vi "Main Dialog.vi"() -> ()   [LabVIEW 2020, in "Process Generation.lvlib" / "New Class Dialog.lvclass"]
uses:
  New Class Dialog.lvclass
  Tag Tree Helper/Tag Tree Helper.lvclass
  Process Generator/Process Generator.lvclass
panel:
  in  "Parent Class":string(tree)
  in  "Process Name":string
  in  "Save to Folder":path
  in  "Commit":bool
  in  "Cancel":bool
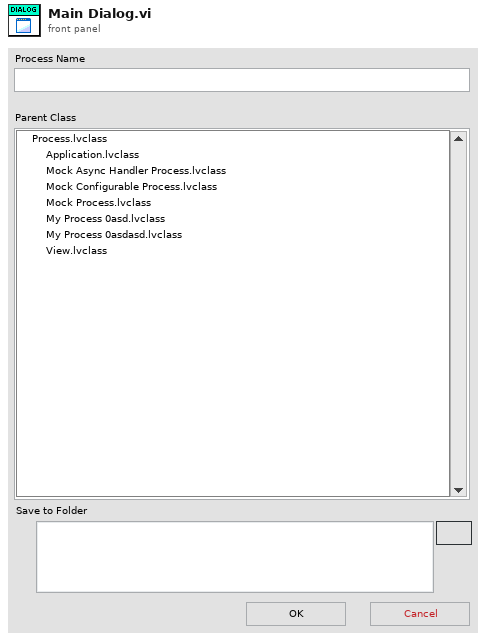
[diagram p1: front panel]
types:
  T1 = enum8{"Enabled", "Disabled", "Disabled and Grayed Out"}
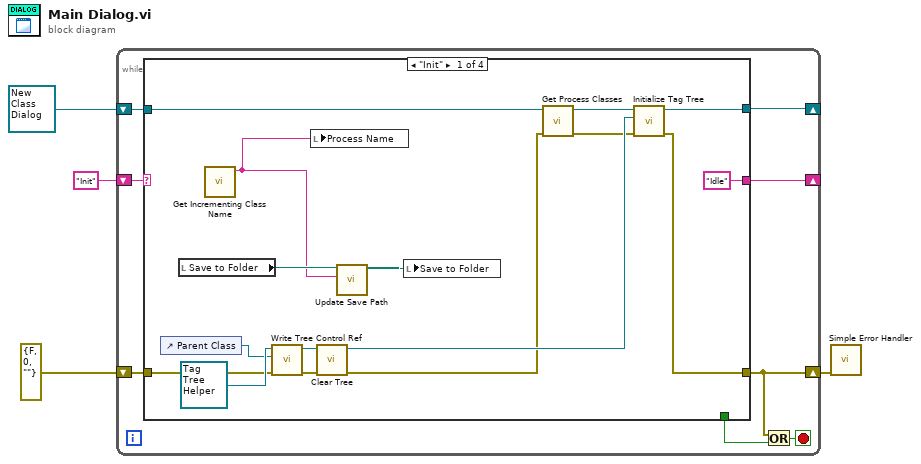
[diagram p0: block diagram]
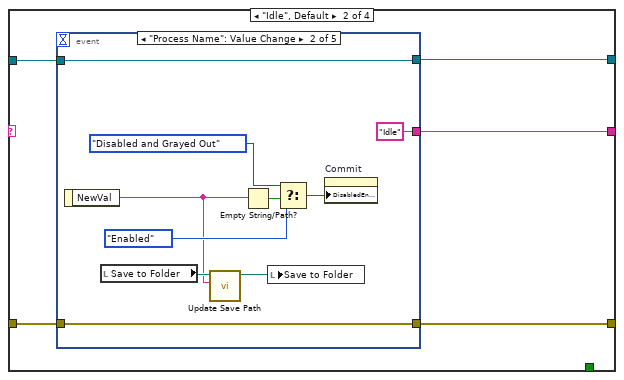
[diagram p2: hidden frame]
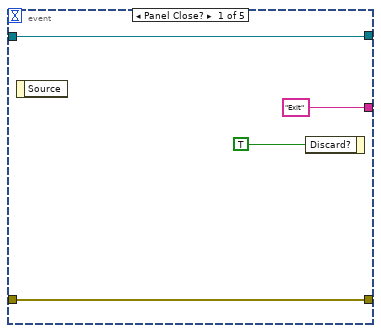
[diagram p3: hidden frame]
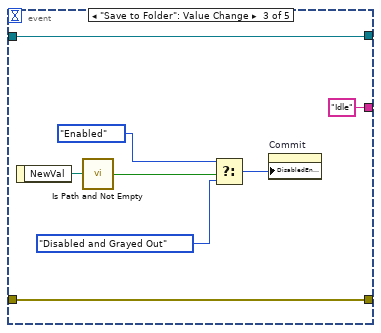
[diagram p4: hidden frame]
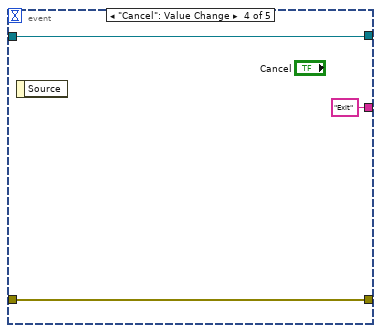
[diagram p5: hidden frame]
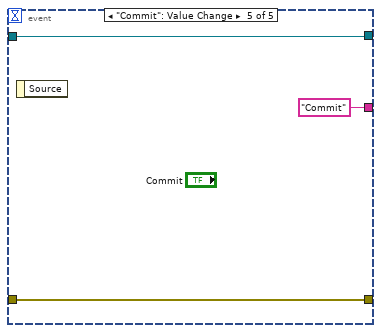
[diagram p6: hidden frame]
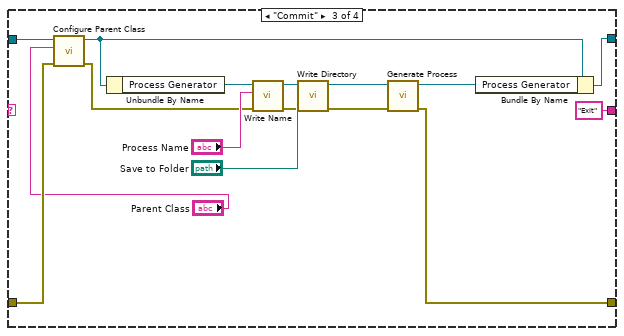
[diagram p7: hidden frame]
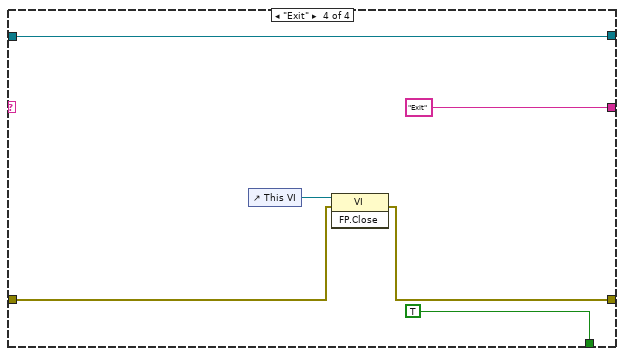
[diagram p8: hidden frame]
diagram:
  n1 = while {
    shift-right: [w9] -> _
    shift-left: refnum<class "New Class Dialog.lvclass"> refnum ("New Class Dialog In") -> [w10]
    shift-right: [w5] -> w2
    shift-left: errorcluster {"status"=FALSE, "code"=0, "source"=""} ("error in (no error)") -> [w11]
    shift-right: [w8] -> _
    shift-left: "Init" -> [w12]
    stop <- w6 stop-if-true
    n2 = case shown="\"Init\"" w12 {
      tunnel: [w22 w33 w64 w79] -> w5
      tunnel: w11 -> [w19 w32 w71 w78]
      tunnel: w10 -> [w27 w31 w68 w83]
      tunnel: [w24 w30 w70 w83] -> w9
      tunnel: ["Idle" w29 "Exit" "Exit"] -> w8
      tunnel: [_ _ _ TRUE] -> w7
      frame "Init" {
        n3 = control-ref of="Parent Class"() -> (w25:refnum<vi>)
        n4 = local read "Save to Folder"() -> (w17:path)
        n5 = call "Get Incrementing Class Name.vi"() -> ("String"=w16:string)  [unwired: 11 in]
        n6 = call "Write Tree Control Ref.vi"("error in (no error)"=w19, "Tag Tree Reference"=w25, "Tag Tree Helper In"=refnum<class "Tag Tree Helper.lvclass"> refnum ("Support Utilities.lvlib:Tag Tree.lvclass")) -> ("error out"=w23:errorcluster, "Tag Tree Helper Out"=w20:refnum<class "Tag Tree Helper.lvclass">)  [unwired: 7 in]
        n7 = local write "Process Name"(w16) -> ()
        n8 = call "Clear Tree.vi"("error in (no error)"=w23, "Tag Tree Helper In"=w20) -> ("error out"=w18:errorcluster, "Tag Tree Helper Out"=w21:refnum<class "Tag Tree Helper.lvclass">)  [unwired: 8 in]
        n9 = call "Update Save Path.vi"("Process Name"=w16, "Current Path"=w17) -> ("Updated Path"=w15:path)  [unwired: 9 in]
        n10 = local write "Save to Folder"(w15) -> ()
        n11 = call "Get Process Classes.vi"("error in (no error)"=w18, "New Class Dialog In"=w27) -> ("error out"=w13:errorcluster, "New Class Dialog Out"=w14:refnum<class "New Class Dialog.lvclass">)  [unwired: 8 in]
        n12 = call "Initialize Tag Tree.vi"("error in (no error)"=w13, "Tag Tree Helper"=w21, "New Class Dialog In"=w14) -> ("error out"=w22:errorcluster, "New Class Dialog Out"=w24:refnum<class "New Class Dialog.lvclass">)  [unwired: 7 in]
      }
      frame "Idle", Default {
        n13 = event shown="[1] \"Process Name\": Value Change" {
          selector: _ -> [_ _ _ _ _]
          dyn-events: _ -> [_ _ _ _ _]
          timeout: _ -> [_ _ _ _ _]
          tunnel: [w37 w47 w55 w57 w61] -> w33
          tunnel: w32 -> [w37 w47 w55 w57 w61]
          tunnel: w31 -> [w36 w46 w54 w58 w60]
          tunnel: [w36 w46 w54 w58 w60] -> w30
          tunnel: ["Exit" "Idle" "Idle" "Exit" "Commit"] -> w29
          event Panel Close? {
            n14 = event-data() -> ()  [unwired: 1 in, 1 out]
            n15 = event-data("Discard?"=TRUE) -> ()  [unwired: 1 in, 1 out]
          }
          event "Process Name": Value Change {
            n16 = event-data() -> ("NewVal"=w38:string)  [unwired: 1 in]
            n17 = local read "Save to Folder"() -> (w39:path)
            n18 = call "Update Save Path.vi"("Process Name"=w38, "Current Path"=w39) -> ("Updated Path"=w40:path)  [unwired: 9 in]
            n19 = Empty String/Path?(string/path=w38) -> (empty?=w45:bool)
            n20 = local write "Save to Folder"(w40) -> ()
            n21 = Select(t=T1."Disabled and Grayed Out" ("Disabled"), s=w45, f=T1."Enabled") -> (s? t:f=w42:T1)
            n22 = property on="Commit" class="Bool"("DisabledEnum"=w42) -> ()  [unwired: 2 in, 2 out]
          }
          event "Save to Folder": Value Change {
            n23 = event-data() -> ("NewVal"=w53:path)  [unwired: 1 in]
            n24 = call <vilib>:"Is Path and Not Empty.vi"("path"=w53) -> ("Is Path and Not Empty?"=w52:bool)  [unwired: 4 in]
            n25 = Select(t=T1."Enabled" ("f"), s=w52, f=T1."Disabled and Grayed Out" ("Disabled")) -> (s? t:f=w49:T1)
            n26 = property on="Commit" class="Bool"("DisabledEnum"=w49) -> ()  [unwired: 2 in, 2 out]
          }
          event "Cancel": Value Change {
            n27 = event-data() -> ()  [unwired: 1 in, 1 out]
          }
          event "Commit": Value Change {
            n28 = event-data() -> ()  [unwired: 1 in, 1 out]
          }
        }
      }
      frame "Commit" {
        n29 = call "Configure Parent Class.vi"("error in (no error)"=w71, "Parent Class"="Parent Class", "New Class Dialog In"=w68) -> ("error out"=w69:errorcluster, "New Class Dialog Out"=w67:refnum<class "New Class Dialog.lvclass">)  [unwired: 7 in]
        n30 = Unbundle By Name(w67) -> ("Process Generator"=w74:refnum<class "Process Generator.lvclass">)
        n31 = call "Write Name.vi"("error in (no error)"=w69, "Name"="Process Name", "Process Generator In"=w74) -> ("error out"=w72:errorcluster, "Process Generator Out"=w73:refnum<class "Process Generator.lvclass">)  [unwired: 7 in]
        n32 = call "Write Directory.vi"("error in (no error)"=w72, "Directory"="Save to Folder", "Process Generator in"=w73) -> ("error out"=w62:errorcluster, "Process Generator out"=w63:refnum<class "Process Generator.lvclass">)  [unwired: 7 in]
        n33 = call "Generate Process.vi"("error in (no error)"=w62, "Process Generator In"=w63) -> ("error out"=w64:errorcluster, "Process Generator Out"=w65:refnum<class "Process Generator.lvclass">)  [unwired: 8 in]
        n34 = Bundle By Name(cluster=w67, "Process Generator"=w65) -> (w70:refnum<class "New Class Dialog.lvclass">)
      }
      frame "Exit" {
        n35 = control-ref of="This VI"() -> (w80:refnum<vi>)
        n36 = invoke class="VI" method="FP.Close"(reference=w80, error in=w78) -> (error out=w79:errorcluster)  [unwired: 1 in, 2 out]
      }
    }
    n37 = Or(x=w5, y=w7) -> (x .or. y?=w6:bool)
  }
  n38 = call <vilib>:"Simple Error Handler.vi"("error in (no error)"=w2) -> ()  [unwired: 4 in, 5 out]
